vi "scale.vi"(10 "dt":dbl=1e-07, 11 "waveforms":dbl[][](array[numeric])=array5x1000[5000 elements]) -> (2 "el":waveform(dbl)[](graph))   [LabVIEW 2013, in "wf_tools.lvlib"]
uses:
  wf_tools.lvlib
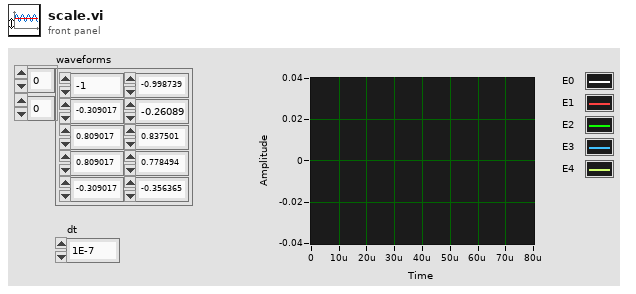
[diagram p1: front panel]
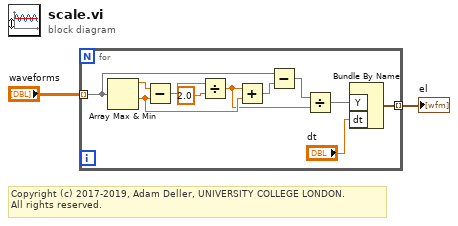
[diagram p0: block diagram]
diagram:
  # "Copyright (c) 2017-2019, Adam Deller, UNIVERSITY COLLEGE LONDON.\nAll rights reserved."
  n1 = for {
    tunnel: "waveforms" -> [w8] mode=indexing
    tunnel: [w4] -> w1 mode=indexing
    n2 = Array Max & Min(array=w8) -> (max value=w11:dbl, min value=w9:dbl)  [unwired: 2 out]
    n3 = Subtract(x=w11, y=w9) -> (x-y=w10:dbl)
    n4 = Divide(x=w10, y=2.0) -> (x/y=w5:dbl)
    n5 = Add(x=w5, y=w9) -> (x+y=w7:dbl)
    n6 = Subtract(x=w8, y=w7) -> (x-y=w6:dbl[])
    n7 = Divide(x=w6, y=w5) -> (x/y=w3:dbl[])
    n8 = Bundle By Name("Y"=w3, "dt"="dt") -> (w4:waveform(dbl))  [unwired: 1 in]
  }
  "el" <- w1
